vi "Send Interface Status.vi"(8 "error in (no error)":errorcluster, 10 "Message":string, 11 "RxTx in":refnum<class "RxTx.lvclass">) -> (0 "error out":errorcluster, 3 "RxTx out":refnum<class "RxTx.lvclass">)   [LabVIEW 2018, in "RxTx.lvclass"]
uses:
  RxTx.lvclass
  RxTx.lvclass/RxTx.ctl
  Interface/Interface.lvclass/Interface.ctl
  Interface/Interface.lvclass
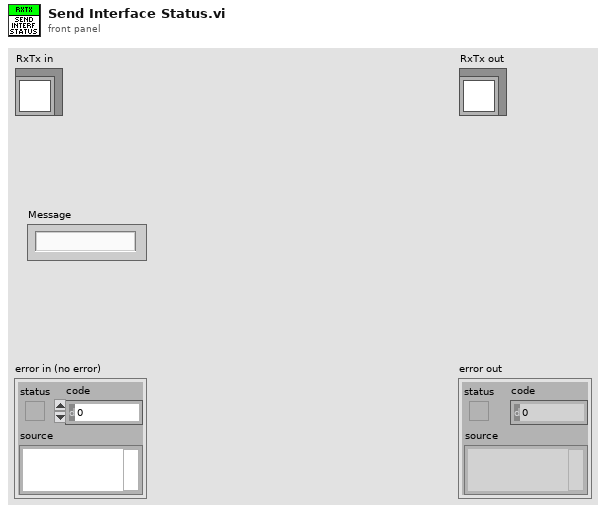
[diagram p1: front panel]
types:
  T1 = cluster{"Current Temperature":i16, "Temperatue Status":string}
  T2 = cluster{"Initialization":bool, "Serial Number":u16}
  T3 = cluster{"Exposure Time":sgl, "Pre-amp gain":u8, "Readout Rate":u8, "EM Mode":u8, "EM Gain":u16, "Binning":u16, "Initial Line":u16, "Initial Cloumn":u16, "Final Line":u16, "Final Column":u16, "Kinetic Series Length":u32, "Shutter Mode":u8, "Cooler ON/OFF":u16, "Temperature":i8, "Image Name":string, "Image Path":string, "#Images":u32}
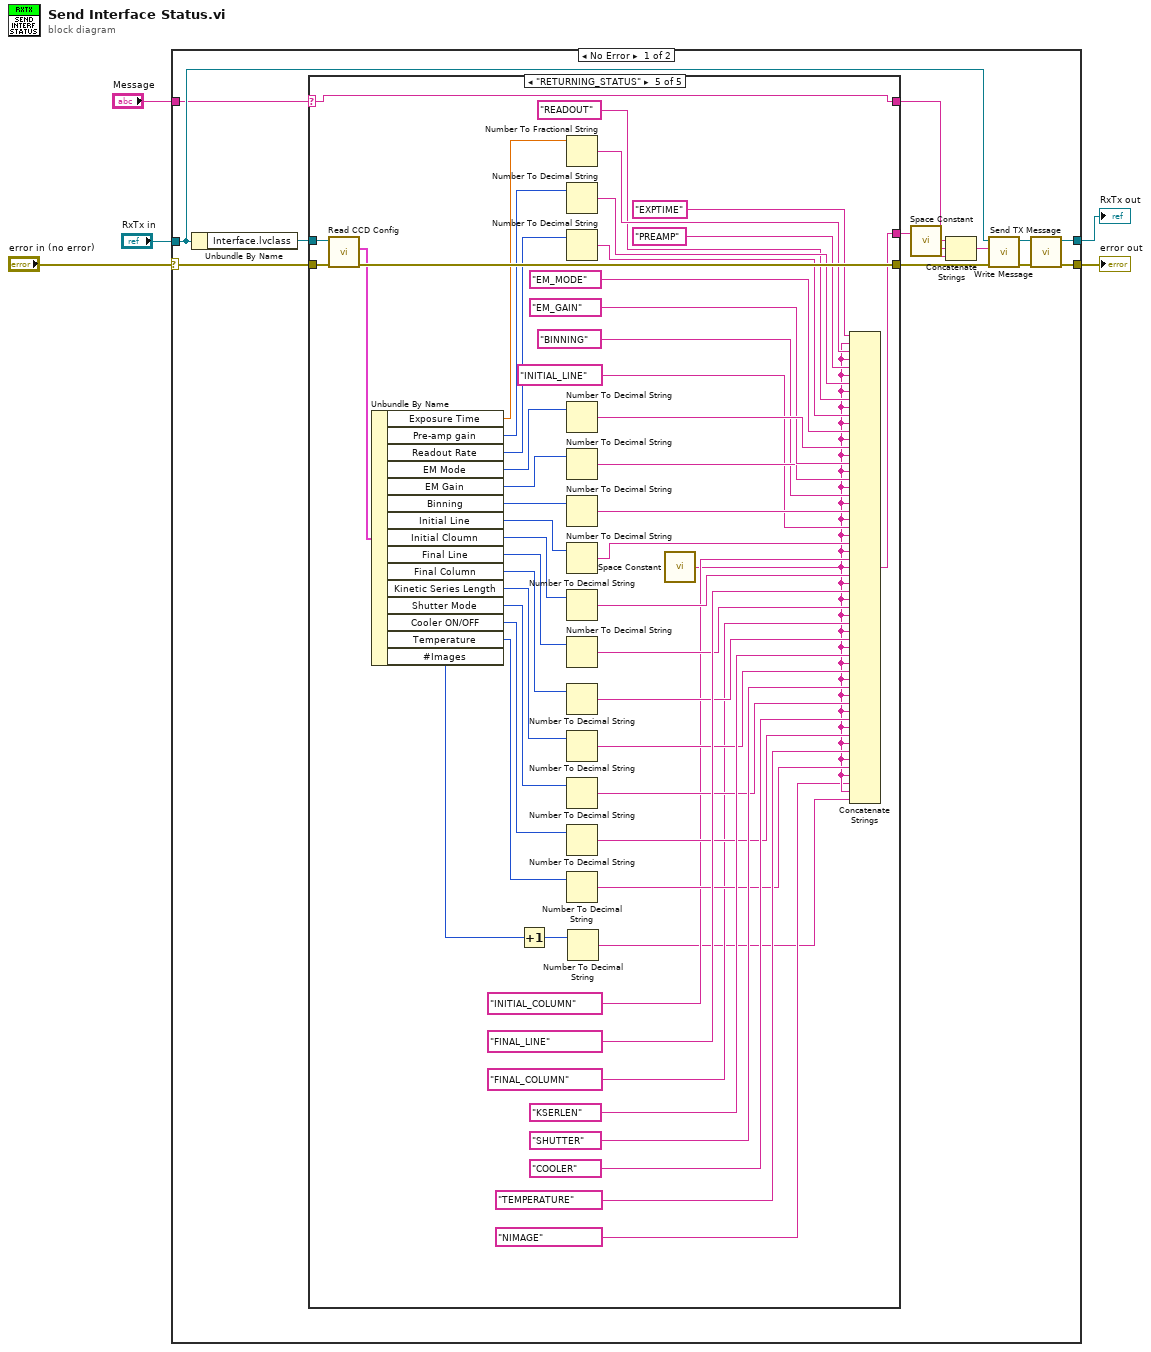
[diagram p0: block diagram]
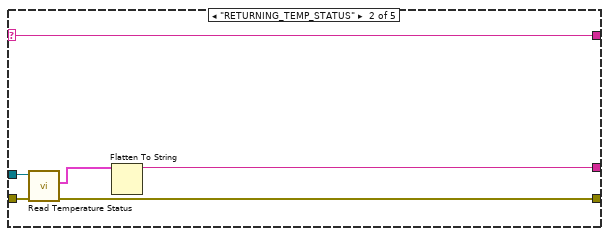
[diagram p3: hidden frame]
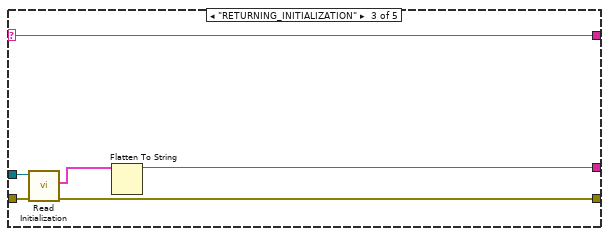
[diagram p4: hidden frame]
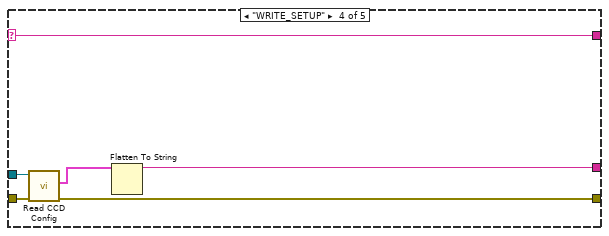
[diagram p5: hidden frame]
diagram:
  n1 = case shown="No Error" "error in (no error)" {
    selector: "error in (no error)" -> [w16 w93]
    tunnel: [w14 w93] -> w2
    tunnel: [w13 w92] -> w1
    tunnel: "RxTx in" -> [w9 w92]
    tunnel: "Message" -> [w6 _]
    frame No Error {
      n2 = Unbundle By Name(w9) -> ("Interface.lvclass"=w18:refnum<class "Interface.lvclass">)
      n3 = case shown="\"RETURNING_STATUS\"" w6 {
        selector: w6 -> [w19 w21 w27 w33 w46]
        tunnel: w18 -> [_ w26 w32 w35 w91]
        tunnel: [w20 w25 w31 w36 w89] -> w11
        tunnel: w16 -> [w20 w24 w30 w37 w90]
        tunnel: [_ w22 w28 w38 w76] -> w15
        tunnel: [w19 w21 w27 w33 w46] -> w7
        frame "False", Default {
        }
        frame "RETURNING_TEMP_STATUS" {
          n4 = call "Read Temperature Status.vi"("error in (no error)"=w24, "Interface in"=w26) -> ("error out"=w25:errorcluster, "Temperature Status"=w23:T1)  [unwired: 7 in, 1 out]
          n5 = Flatten To String(anything=w23) -> (data string=w22:string)  [unwired: 3 in, 2 out]
        }
        frame "RETURNING_INITIALIZATION" {
          n6 = call "Read Initialization.vi"("error in (no error)"=w30, "Interface in"=w32) -> ("error out"=w31:errorcluster, "Initialization"=w29:T2)  [unwired: 7 in, 1 out]
          n7 = Flatten To String(anything=w29) -> (data string=w28:string)  [unwired: 3 in, 2 out]
        }
        frame "WRITE_SETUP" {
          n8 = call "Read CCD Config.vi"("error in (no error)"=w37, "Interface in"=w35) -> ("error out"=w36:errorcluster, "CCD Config"=w34:T3)  [unwired: 7 in, 1 out]
          n9 = Flatten To String(anything=w34) -> (data string=w38:string)  [unwired: 3 in, 2 out]
        }
        frame "RETURNING_STATUS" {
          n10 = call "Read CCD Config.vi"("error in (no error)"=w90, "Interface in"=w91) -> ("error out"=w89:errorcluster, "CCD Config"=w88:T3)  [unwired: 7 in, 1 out]
          n11 = Unbundle By Name(w88) -> ("Exposure Time"=w85:sgl, "Pre-amp gain"=w84:u8, "Readout Rate"=w83:u8, "EM Mode"=w82:u8, "EM Gain"=w81:u16, "Binning"=w71:u16, "Initial Line"=w68:u16, "Initial Cloumn"=w65:u16, "Final Line"=w62:u16, "Final Column"=w60:u16, "Kinetic Series Length"=w58:u32, "Shutter Mode"=w55:u8, "Cooler ON/OFF"=w51:u16, "Temperature"=w48:i8, "#Images"=w39:u32)
          n12 = Increment(x=w39) -> (x+1=w40:u32)
          n13 = Number To Fractional String(number=w85) -> (F-format string=w86:string)  [unwired: 3 in]
          n14 = Number To Decimal String(number=w84) -> (decimal integer string=w79:string)  [unwired: 1 in]
          n15 = Number To Decimal String(number=w83) -> (decimal integer string=w77:string)  [unwired: 1 in]
          n16 = Number To Decimal String(number=w82) -> (decimal integer string=w74:string)  [unwired: 1 in]
          n17 = Number To Decimal String(number=w81) -> (decimal integer string=w72:string)  [unwired: 1 in]
          n18 = Number To Decimal String(number=w71) -> (decimal integer string=w69:string)  [unwired: 1 in]
          n19 = Number To Decimal String(number=w68) -> (decimal integer string=w66:string)  [unwired: 1 in]
          n20 = Number To Decimal String(number=w65) -> (decimal integer string=w64:string)  [unwired: 1 in]
          n21 = Number To Decimal String(number=w62) -> (decimal integer string=w61:string)  [unwired: 1 in]
          n22 = Number To Decimal String(number=w60) -> (decimal integer string=w59:string)  [unwired: 1 in]
          n23 = Number To Decimal String(number=w58) -> (decimal integer string=w56:string)  [unwired: 1 in]
          n24 = Number To Decimal String(number=w55) -> (decimal integer string=w53:string)  [unwired: 1 in]
          n25 = Number To Decimal String(number=w51) -> (decimal integer string=w50:string)  [unwired: 1 in]
          n26 = Number To Decimal String(number=w48) -> (decimal integer string=w47:string)  [unwired: 1 in]
          n27 = Number To Decimal String(number=w40) -> (decimal integer string=w41:string)  [unwired: 1 in]
          n28 = call <vilib>:"Space Constant.vi"() -> ("String"=w43:string)
          n29 = Concatenate Strings("EXPTIME", w43, w86, w43, "PREAMP", w43, w79, w43, "READOUT", w43, w77, w43, "EM_MODE", w43, w74, w43, "EM_GAIN", w43, w72, w43, "BINNING", w43, w69, w43, "INITIAL_LINE", w43, w66, w43, "INITIAL_COLUMN", w43, w64, w43, "FINAL_LINE", w43, w61, w43, "FINAL_COLUMN", w43, w59, w43, "KSERLEN", w43, w56, w43, "SHUTTER", w43, w53, w43, "COOLER", w43, w50, w43, "TEMPERATURE", w43, w47, w43, "NIMAGE", w43, w41) -> (w76:string)
        }
      }
      n30 = call <vilib>:"Space Constant.vi"() -> ("String"=w17:string)
      n31 = Concatenate Strings(w7, w17, w15) -> (w10:string)
      n32 = call "Write Message.vi"("error in (no error)"=w11, "Message"=w10, "RxTx in"=w9) -> ("error out"=w12:errorcluster, "RxTx out"=w8:refnum<class "RxTx.lvclass">)  [unwired: 7 in]
      n33 = call "Send TX Message.vi"("error in (no error)"=w12, "RxTx in"=w8) -> ("error out"=w14:errorcluster, "RxTx out"=w13:refnum<class "RxTx.lvclass">)  [unwired: 8 in]
    }
    frame Error {
    }
  }
  "error out" <- w2
  "RxTx out" <- w1
